vi "DMS_load_sample_BM.vi"(6 "COM Port":refnum<visa-resource-name>="COM9", 7 "Pump Parameters":T2={"Speed 1"="100", "Speed 2"="250", "Speed 3"="250", "Speed 4"="250", "UW/Sample"="5", "Sparge"="2", "Std"="4", "Waste"="15", "Air"="14", "Milli-Q"="1", "H2SO4"="6", "NaOH"="3", "Catalyst"="7", "Cell (H+ side)"="8", "Cell (sample side)"="9", "NaCl"="9"}, 8 "Mode Selection":T1(ring), 9 "step to ml":dbl=1920.0, 10 "Total Vol. (mL)":dbl, 11 "Sample Vol. (mL)":dbl=10.0) -> ()   [LabVIEW 2021]
panel:
  out "Full Command":string="o4A0V5000o1P14400o4D14400o1P33600o4D9600o2D24000o5P9600o2D9600o6P33600o4D33600"
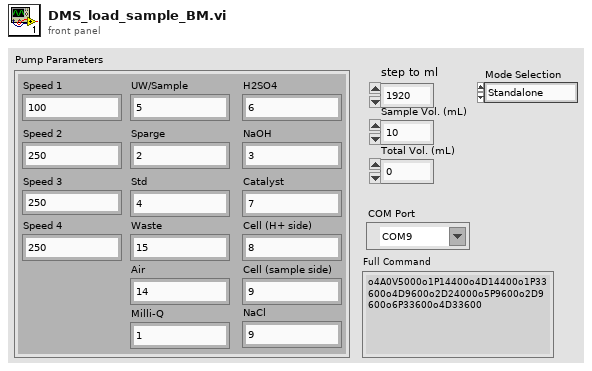
[diagram p1: front panel]
types:
  T1 = enum16{"Standalone", "Standard Curve", "Point Std", "Analysis"}
  T2 = cluster{"Speed 1":string, "Speed 2":string, "Speed 3":string, "Speed 4":string, "UW/Sample":string, "Sparge":string, "Std":string, "Waste":string, "Air":string, "Milli-Q":string, "H2SO4":string, "NaOH":string, "Catalyst":string, "Cell (H+ side)":string, "Cell (sample side)":string, "NaCl":string}
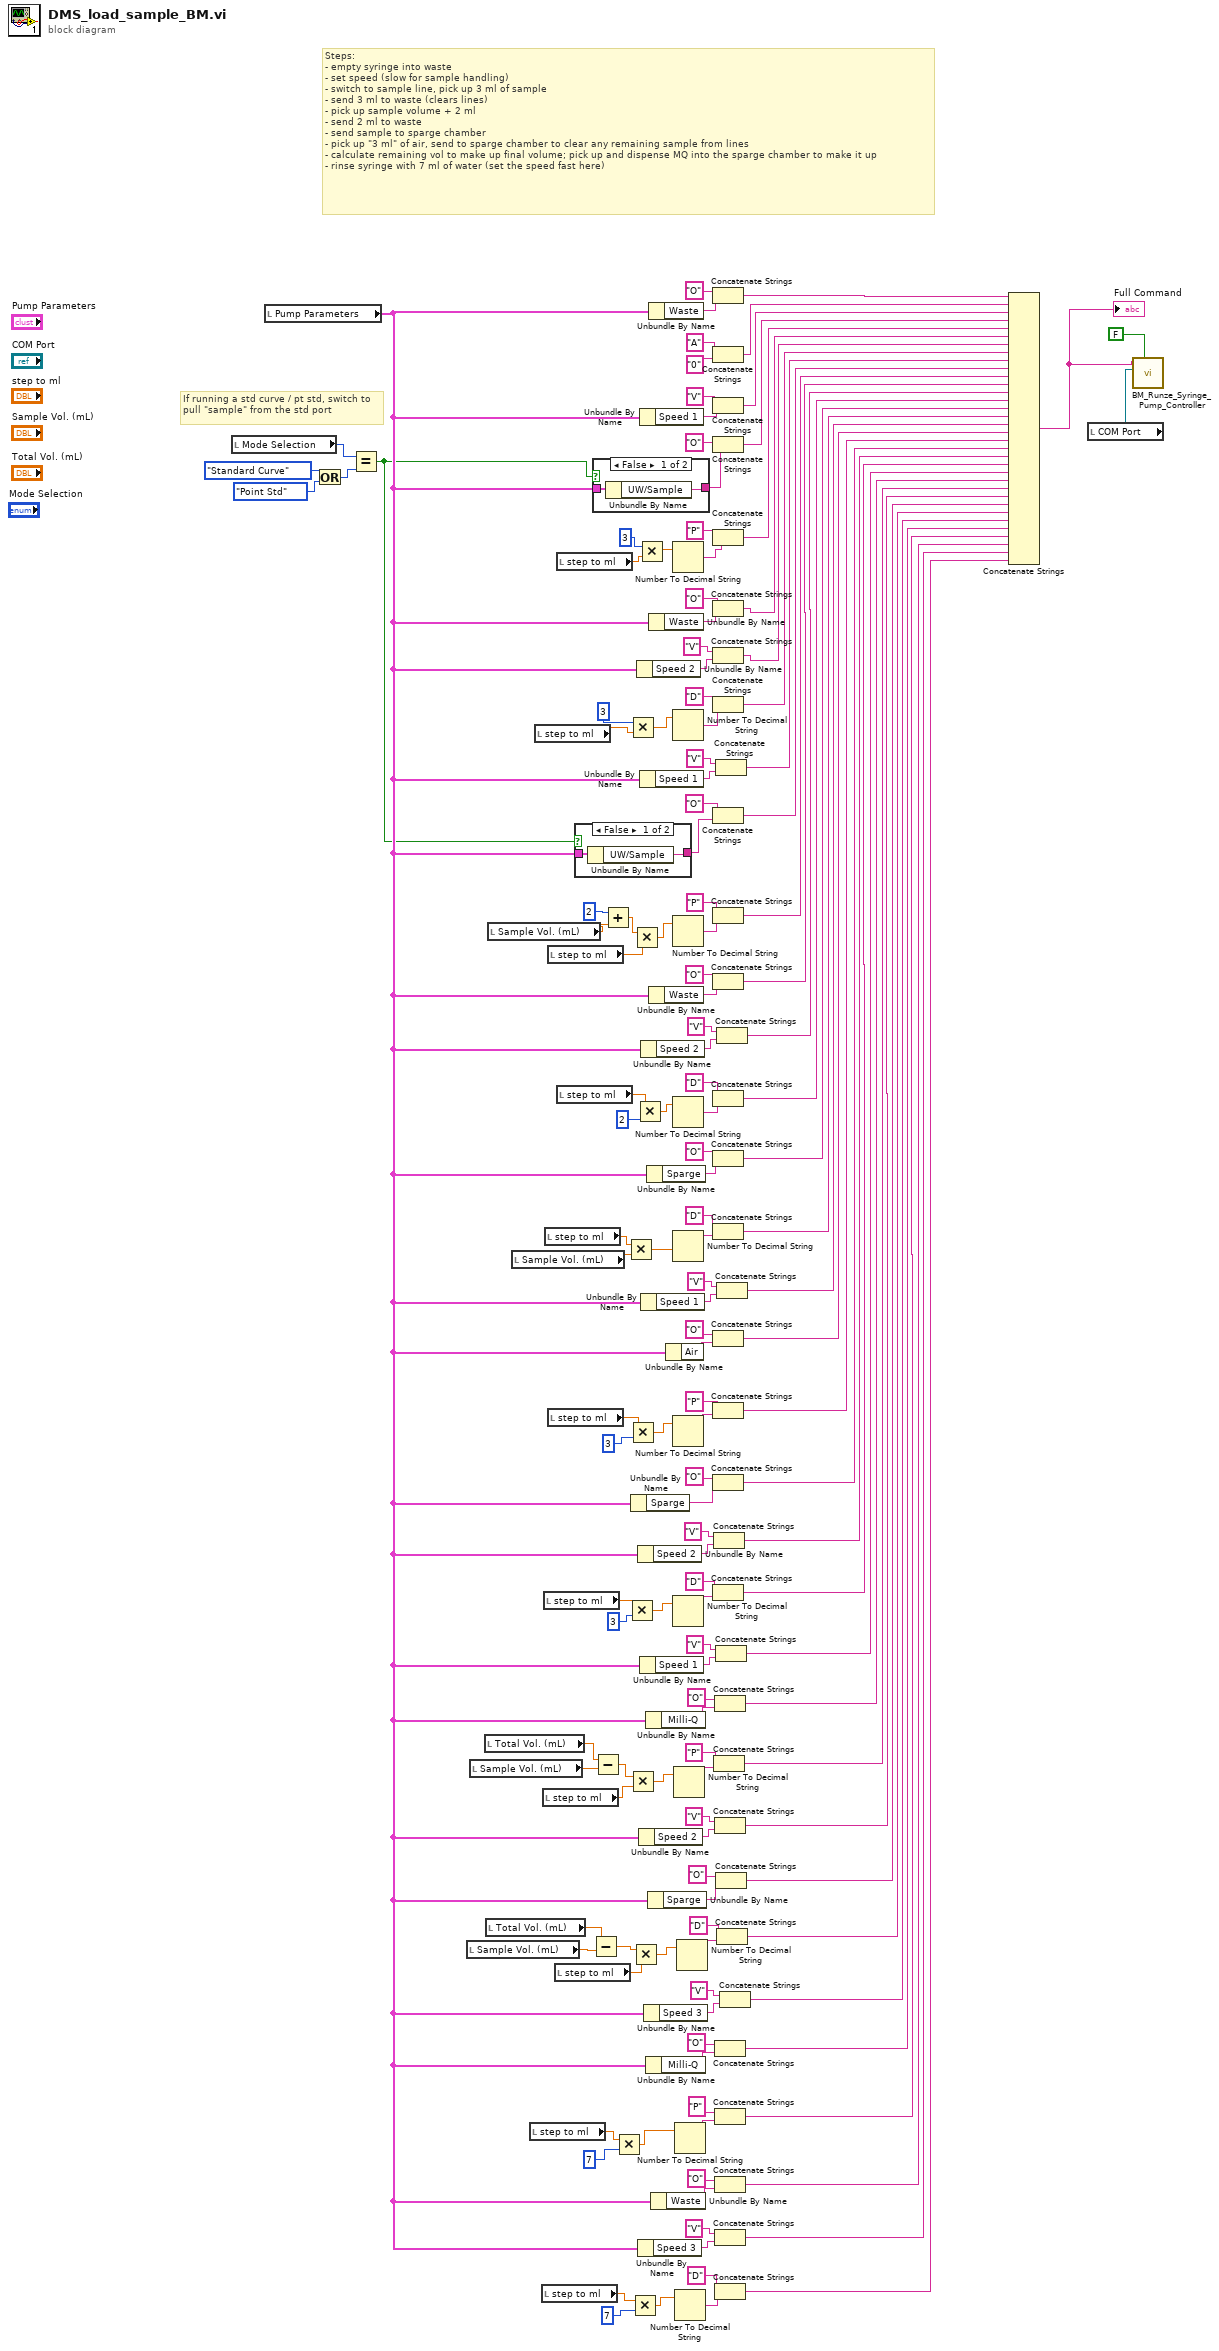
[diagram p0: block diagram]
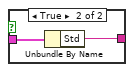
[diagram p2: hidden frame]
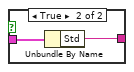
[diagram p3: hidden frame]
diagram:
  # "If running a std curve / pt std, switch to pull \"sample\" from the std port"
  # "Steps:\n- empty syringe into waste\n- set speed (slow for sample handling)\n- switch to sample line, pick up 3 ml of sample\n- send 3 ml to waste (clears lines)\n- pick up sample volume + 2 ml\n- send 2 ml to waste\n- send sample to sparge chamber\n- pick up \"3 ml\" of air, send to sparge chamber to clear any remaining sample from lines\n- calculate remaining vol to make up final volume; pick up and dispense MQ into the sparge chamber to make it up\n- rinse syringe with 7 ml of water (set the speed fast here)"
  n1 = local read "Mode Selection"() -> (w9:T1)
  n2 = local read "Pump Parameters"() -> (w5:T2)
  n3 = Or(x=T1."Standard Curve" ("y"), y=T1."Point Std") -> (x .or. y?=w6:i32)
  n4 = Equal?(x=w9, y=w6) -> (x = y?=w3:bool)
  n5 = local read "Sample Vol. (mL)"() -> (w2:dbl)
  n6 = local read "Sample Vol. (mL)"() -> (w1:dbl)
  n7 = local read "Total Vol. (mL)"() -> (w29:dbl)
  n8 = local read "Total Vol. (mL)"() -> (w28:dbl)
  n9 = local read "Sample Vol. (mL)"() -> (w109:dbl)
  n10 = local read "Sample Vol. (mL)"() -> (w108:dbl)
  n11 = local read "step to ml"() -> (w120:dbl)
  n12 = local read "step to ml"() -> (w103:dbl)
  n13 = local read "step to ml"() -> (w83:dbl)
  n14 = local read "step to ml"() -> (w35:dbl)
  n15 = local read "step to ml"() -> (w92:dbl)
  n16 = local read "step to ml"() -> (w122:dbl)
  n17 = local read "step to ml"() -> (w123:dbl)
  n18 = local read "step to ml"() -> (w121:dbl)
  n19 = local read "step to ml"() -> (w26:dbl)
  n20 = local read "step to ml"() -> (w125:dbl)
  n21 = local read "step to ml"() -> (w124:dbl)
  n22 = case shown="False" w3 {
    tunnel: [w151 w154] -> w4
    tunnel: w5 -> [w152 w153]
    frame False {
      n23 = Unbundle By Name(w152) -> ("UW/Sample"=w151:string)
    }
    frame True {
      n24 = Unbundle By Name(w153) -> ("Std"=w154:string)
    }
  }
  n25 = Subtract(x=w28, y=w2) -> (x-y=w27:dbl)
  n26 = case shown="False" w3 {
    tunnel: [w155 w158] -> w117
    tunnel: w5 -> [w156 w157]
    frame False {
      n27 = Unbundle By Name(w156) -> ("UW/Sample"=w155:string)
    }
    frame True {
      n28 = Unbundle By Name(w157) -> ("Std"=w158:string)
    }
  }
  n29 = Subtract(x=w29, y=w1) -> (x-y=w36:dbl)
  n30 = Add(x=2, y=w109) -> (x+y=w143:dbl)
  n31 = Multiply(x=w120, y=7) -> (x*y=w140:dbl)
  n32 = Multiply(x=w122, y=w108) -> (x*y=w147:dbl)
  n33 = Multiply(x=w92, y=3) -> (x*y=w93:dbl)
  n34 = Multiply(x=3, y=w103) -> (x*y=w104:dbl)
  n35 = Multiply(x=w121, y=3) -> (x*y=w146:dbl)
  n36 = Multiply(x=w36, y=w35) -> (x*y=w39:dbl)
  n37 = Multiply(x=w83, y=7) -> (x*y=w85:dbl)
  n38 = Unbundle By Name(w5) -> ("Sparge"=w112:string)
  n39 = Multiply(x=w27, y=w26) -> (x*y=w32:dbl)
  n40 = Multiply(x=w143, y=w123) -> (x*y=w144:dbl)
  n41 = Multiply(x=w124, y=2) -> (x*y=w149:dbl)
  n42 = Multiply(x=3, y=w125) -> (x*y=w141:dbl)
  n43 = Unbundle By Name(w5) -> ("Speed 2"=w78:string)
  n44 = Unbundle By Name(w5) -> ("Speed 2"=w70:string)
  n45 = Unbundle By Name(w5) -> ("Speed 3"=w21:string)
  n46 = Unbundle By Name(w5) -> ("Speed 2"=w24:string)
  n47 = Unbundle By Name(w5) -> ("Speed 1"=w118:string)
  n48 = Unbundle By Name(w5) -> ("Speed 1"=w77:string)
  n49 = Unbundle By Name(w5) -> ("Speed 1"=w69:string)
  n50 = Unbundle By Name(w5) -> ("Speed 2"=w74:string)
  n51 = Unbundle By Name(w5) -> ("Speed 1"=w73:string)
  n52 = Unbundle By Name(w5) -> ("Speed 3"=w23:string)
  n53 = Unbundle By Name(w5) -> ("Milli-Q"=w40:string)
  n54 = Unbundle By Name(w5) -> ("Milli-Q"=w111:string)
  n55 = Unbundle By Name(w5) -> ("Sparge"=w114:string)
  n56 = Unbundle By Name(w5) -> ("Sparge"=w33:string)
  n57 = Unbundle By Name(w5) -> ("Waste"=w119:string)
  n58 = Unbundle By Name(w5) -> ("Waste"=w116:string)
  n59 = Unbundle By Name(w5) -> ("Waste"=w115:string)
  n60 = Unbundle By Name(w5) -> ("Waste"=w110:string)
  n61 = Unbundle By Name(w5) -> ("Air"=w113:string)
  n62 = Number To Decimal String(number=w141) -> (decimal integer string=w102:string)  [unwired: 1 out]
  n63 = Number To Decimal String(number=w104) -> (decimal integer string=w101:string)  [unwired: 1 out]
  n64 = Number To Decimal String(number=w144) -> (decimal integer string=w99:string)  [unwired: 1 out]
  n65 = Number To Decimal String(number=w149) -> (decimal integer string=w98:string)  [unwired: 1 out]
  n66 = Number To Decimal String(number=w147) -> (decimal integer string=w95:string)  [unwired: 1 out]
  n67 = Number To Decimal String(number=w146) -> (decimal integer string=w90:string)  [unwired: 1 out]
  n68 = Number To Decimal String(number=w93) -> (decimal integer string=w88:string)  [unwired: 1 out]
  n69 = Number To Decimal String(number=w39) -> (decimal integer string=w37:string)  [unwired: 1 out]
  n70 = Number To Decimal String(number=w140) -> (decimal integer string=w86:string)  [unwired: 1 out]
  n71 = Number To Decimal String(number=w85) -> (decimal integer string=w82:string)  [unwired: 1 out]
  n72 = Number To Decimal String(number=w32) -> (decimal integer string=w30:string)  [unwired: 1 out]
  n73 = Concatenate Strings("O", w119) -> (w65:string)
  n74 = Concatenate Strings("A", "0") -> (w64:string)
  n75 = Concatenate Strings("V", w118) -> (w63:string)
  n76 = Concatenate Strings("O", w117) -> (w62:string)
  n77 = Concatenate Strings("P", w102) -> (w61:string)
  n78 = Concatenate Strings("O", w116) -> (w60:string)
  n79 = Concatenate Strings("V", w78) -> (w59:string)
  n80 = Concatenate Strings("D", w101) -> (w58:string)
  n81 = Concatenate Strings("O", w4) -> (w56:string)
  n82 = Concatenate Strings("P", w99) -> (w55:string)
  n83 = Concatenate Strings("O", w115) -> (w54:string)
  n84 = Concatenate Strings("D", w98) -> (w52:string)
  n85 = Concatenate Strings("O", w114) -> (w51:string)
  n86 = Concatenate Strings("D", w95) -> (w50:string)
  n87 = Concatenate Strings("O", w113) -> (w48:string)
  n88 = Concatenate Strings("P", w90) -> (w47:string)
  n89 = Concatenate Strings("O", w112) -> (w46:string)
  n90 = Concatenate Strings("D", w88) -> (w44:string)
  n91 = Concatenate Strings("V", w70) -> (w45:string)
  n92 = Concatenate Strings("P", w37) -> (w19:string)
  n93 = Concatenate Strings("O", w40) -> (w20:string)
  n94 = Concatenate Strings("V", w24) -> (w18:string)
  n95 = Concatenate Strings("O", w111) -> (w14:string)
  n96 = Concatenate Strings("P", w86) -> (w13:string)
  n97 = Concatenate Strings("O", w110) -> (w12:string)
  n98 = Concatenate Strings("V", w21) -> (w11:string)
  n99 = Concatenate Strings("D", w82) -> (w10:string)
  n100 = Concatenate Strings("V", w77) -> (w57:string)
  n101 = Concatenate Strings("V", w69) -> (w43:string)
  n102 = Concatenate Strings("O", w33) -> (w17:string)
  n103 = Concatenate Strings("V", w74) -> (w53:string)
  n104 = Concatenate Strings("V", w73) -> (w49:string)
  n105 = Concatenate Strings("D", w30) -> (w16:string)
  n106 = Concatenate Strings("V", w23) -> (w15:string)
  n107 = Concatenate Strings(w65, w64, w63, w62, w61, w60, w59, w58, w57, w56, w55, w54, w53, w52, w51, w50, w49, w48, w47, w46, w45, w44, w43, w20, w19, w18, w17, w16, w15, w14, w13, w12, w11, w10) -> (w128:string)
  "Full Command" <- w128
  n108 = local read "COM Port"() -> (w127:refnum<visa-resource-name>)
  n109 = call "BM_Runze_Syringe_Pump_Controller.vi"("Initialize Plunger?"=FALSE ("Initialize?"), "COM Port (Runze)"=w127, "Enter Command"=w128) -> ()  [unwired: 6 in, 3 out]
